vi "shake it.vi"(4 "cursor bracket : fragment 2":refnum<vi>, 5 "modify if out of window?":bool=TRUE, 6 "cursor bracket: All, data window 2":refnum<vi>, 7 "Plot: All":refnum<vi>, 8 "follow the peak Con":T1={"factor"=3.0, "omega ?"=TRUE, "gamma ?"=TRUE, "max (kHz)"=3.0, "is clean"=TRUE, "acceptance"=0.3, "history - length"=10}, 9 "search attempts":i32=4, 10 "peak close to center -- factor":dbl=0.3, 11 "lorentzian":T3={"Amplitude"=0.005126003617902175, "omega(0)"=2152.184993711879, "Gamma"=1.6893036092699798, "phase"=-0.5171067718590723, "Q"=1274.0072192481316, "Norm  Ampl"=0.7704795248463377, "z (inf)"=0.18381077367248932+0.35479358908517594i, "4corners"={"z (-pi/2)"=0.35479358908517594-0.2671441070058228i, "z(inf)"=0.18381077367248932+0.35479358908517594i, "z (pi/2)"=-0.4381269224185094+0.18381077367248932i, "z center"=-0.04166666666666674-0.04166666666666674i, "z(0)"=-0.2671441070058228-0.4381269224185094i, "radius"=0.4560929844809216}} {"z (inf)" format="%#9_9f"; "Q" format="%#9_9f"; "phase" format="%#9_9f"; "Gamma" format="%#9_9f"; "omega(0)" format="%#9_9f"}) -> (0 "Boolean":bool, 1 "worth trying":bool, 2 "in range?":bool=TRUE, 3 "lorentzian out":T3={"Amplitude"=0.005126003617902175, "omega(0)"=2152.184993711879, "Gamma"=1.6893036092699798, "phase"=-0.5171067718590723, "Q"=1274.0072192481316, "Norm  Ampl"=0.7704795248463377, "z (inf)"=0.18381077367248932+0.35479358908517594i, "4corners"={"z (-pi/2)"=0.35479358908517594-0.2671441070058228i, "z(inf)"=0.18381077367248932+0.35479358908517594i, "z (pi/2)"=-0.4381269224185094+0.18381077367248932i, "z center"=-0.04166666666666674-0.04166666666666674i, "z(0)"=-0.2671441070058228-0.4381269224185094i, "radius"=0.4560929844809216}} {"z (inf)" format="%#9_9f"; "Q" format="%#9_9f"; "phase" format="%#9_9f"; "Gamma" format="%#9_9f"; "omega(0)" format="%#9_9f"})   [LabVIEW 2015]
uses:
  lorentzian.ctl
  circle corners.ctl
  cursor winow.ctl
  follow the peak control.ctl
  cursor window action.ctl
panel:
  in  "cursor bracket in":T2={"left"=2044.0881763527054, "right "=2126.7657992565055, "center"=2085.4269878046052, "window"=82.67762290380006, "cursors"=[], "relative"=0, "absolute"=0, "fixed vertical offset"=2421.6740576496672, "vertical offset"=2421.6740576496672, "skew"=2421.6740576496672, "default window frac"=2421.6740576496672, "kind"=enum."fancy", "skew.left"=2.0, "skew.right"=0.0, "Plot ref"=refnum, "wing order"=enum."back"}
  in  "follow the peak is clean -- out":bool
  out "attempts to success":i32
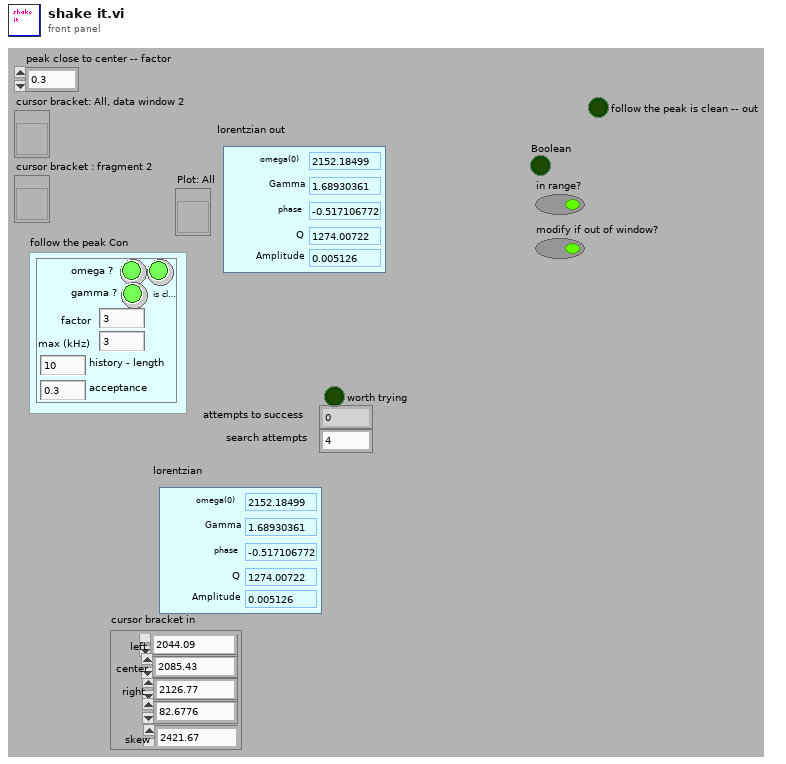
[diagram p1: front panel]
types:
  T1 = typedef "follow the peak control.ctl" = cluster{"factor":dbl, "omega ?":bool, "gamma ?":bool, "max (kHz)":dbl, "is clean":bool, "acceptance":dbl, "history - length":i32}
  T2 = typedef "cursor winow.ctl" = cluster{"left":dbl, "right ":dbl, "center":dbl, "window":dbl, "cursors":i32[], "relative":i32, "absolute":i32, "fixed vertical offset":dbl, "vertical offset":dbl, "skew":dbl, "default window frac":dbl, "kind":enum16{"symmetric", "skewed", "fancy"}, "skew.left":dbl, "skew.right":dbl, "Plot ref":refnum<vi>, "wing order":enum16{"forw", "back"}}
  T3 = typedef "lorentzian.ctl" = cluster{"Amplitude":dbl, "omega(0)":dbl, "Gamma":dbl, "phase":dbl, "Q":dbl, "Norm  Ampl":dbl, "z (inf)":cdb, "4corners":T4}
  T4 = typedef "circle corners.ctl" = cluster{"z (-pi/2)":cdb, "z(inf)":cdb, "z (pi/2)":cdb, "z center":cdb, "z(0)":cdb, "radius":dbl}
  T5 = typedef "cursor window action.ctl" = enum16{"balance", "h. offset change", "cursor moves", "change center", "change window", "init", "check", "reset", "set y to middle", "idle", "-write all Y", "-write left.X", "-write center.X", "-write right.X", "-write all X", "-change center", "-change window", "-change skew", "-read cursor 2", "-read cursor 1", "-read cursor 0", "-read all cursors", "-reset", "-read plot scale", "-set y to middle", "-Q: center.Y is visible", "-Q: window is visible", "-parse center.Y", "-right left from center", "-left move", "-right move", "-set center.Y", "-empty", "-set cursors to default", "-check", "-write center.Y", "-copy cursor 1", "-copy cursor 0", "-copy cursor 2", "move right", "move left", "shrink", "broaden", "skew up", "skew down", "-write plot scale", "zoom X", "change cen&win", "zoom to all data"}
  T6 = enum16{"normal", "alert", "fuzzy", "interesting", "boring", "colored"}
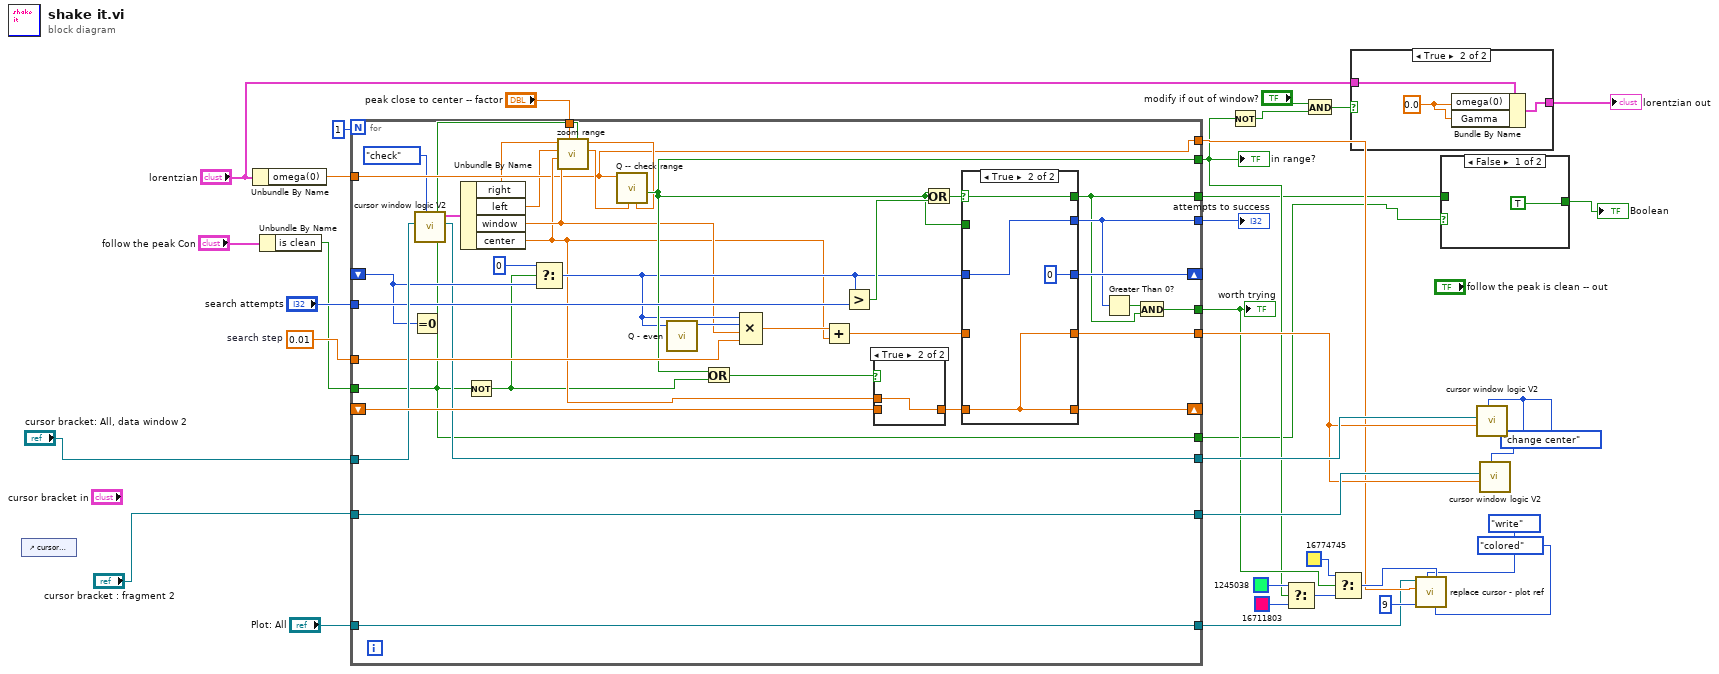
[diagram p0: block diagram]
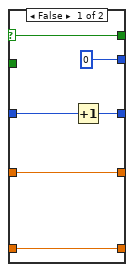
[diagram p5: hidden frame]
diagram:
  w5 = cursor_window_action."change center" ("cursor window action")
  w30 = 0.01  # search step
  n1 = control-ref of="cursor bracket in"() -> ()  [unwired: 1 out]
  n2 = Unbundle By Name("lorentzian") -> ("omega(0)"=w33:dbl)
  n3 = Unbundle By Name("follow the peak Con") -> ("is clean"=w1:bool)
  n4 = for {
    N: 1 -> [_]
    shift-right: [w72] -> _
    shift-left: _ -> [w51]
    shift-right: [w70] -> _
    shift-left: _ -> [w69]
    tunnel: "Plot: All" -> [w47]
    tunnel: "cursor bracket: All, data window 2" -> [w62]
    tunnel: w33 -> [w42]
    tunnel: [w57] -> w6
    tunnel: "cursor bracket : fragment 2" -> [w49]
    tunnel: [w58] -> w32
    tunnel: [w54] -> w10
    tunnel: "search attempts" -> [w61]
    tunnel: w30 -> [w60]
    tunnel: [w56] -> w13
    tunnel: w1 -> [w40]
    tunnel: [w50] -> w24
    tunnel: [w49] -> w23
    tunnel: [w48] -> w22
    tunnel: [w42] -> w12
    tunnel: [w47] -> w11
    tunnel: [w40] -> w8
    tunnel: "peak close to center -- factor" -> [w41]
    n5 = Equal To 0?(x=w51) -> ()  [unwired: 1 out]
    n6 = call "cursor window logic V2.vi"("cursor window action"=cursor_window_action."check", "cursor window in"=w62) -> (2:"cursor window out"=w50:refnum<vi>, 3:"cursor window out"=w68:T2)  [unwired: 8 in]
    n7 = Unbundle By Name(w68) -> ("right"=w39:dbl, "left"=w38:dbl, "window"=w46:dbl, "center"=w45:dbl)
    n8 = Not(x=w40) -> (.not. x?=w37:bool)
    n9 = Select(t=0 ("interval"), s=w37, f=w51) -> (s? t:f=w53:i32)
    n10 = call "zoom range.vi"("zoom?"=w40, "factor"=w41, "window"=w46, "center"=w45, "left"=w38, "right"=w39) -> ("left out"=w44:dbl, "right out"=w43:dbl)  [unwired: 2 in, 2 out]
    n11 = call "Q -- check range.vi"("upper"=w43, "lower"=w44, "number"=w42) -> ("in range?"=w54:bool)  [unwired: 4 in, 4 out]
    n12 = call "Q - even.vi"("Numeric"=w53) -> ("saw"=w66:i32)  [unwired: 9 in, 1 out]
    n13 = Or(x=w54, y=w37) -> (x .or. y?=w55:bool)
    n14 = Compound Arithmetic op=MULTIPLY(w53, w66, w46, w60) -> (w67:dbl)
    n15 = Add(x=w67, y=w45) -> (x+y=w71:dbl)
    n16 = Greater?(x=w53, y=w61) -> (0:w64:bool)
    n17 = case shown="True" w55 {
      tunnel: [w73 w74] -> w63
      tunnel: w45 -> [_ w74]
      tunnel: w69 -> [w73 _]
      frame False {
      }
      frame True {
      }
    }
    n18 = Or(x=w54, y=w64) -> (x .or. y?=w65:bool)
    n19 = case shown="True" w65 {
      selector: w65 -> [w77 w83]
      tunnel: [w79 0 ("interval")] -> w72
      tunnel: w53 -> [w80 w82]
      tunnel: w71 -> [w75 _]
      tunnel: [w78 w81] -> w70
      tunnel: w63 -> [w78 w81]
      tunnel: w54 -> [_ _]
      tunnel: [w77 w83] -> w57
      tunnel: [0 ("interval") w82] -> w58
      tunnel: [w75 w81] -> w48
      frame False {
        n20 = Increment(x=w80) -> (x+1=w79:i32)
      }
      frame True {
      }
    }
    n21 = Greater Than 0?(x=w58) -> (x > 0?=w59:bool)
    n22 = And(x=w59, y=w57) -> (x .and. y?=w56:bool)
  }
  "attempts to success" <- w32
  "in range?" <- w10
  "worth trying" <- w13
  n23 = Not(x=w10) -> (.not. x?=w29:bool)
  n24 = Select(t=u32 1245038, s=w10, f=u32 16711803) -> (s? t:f=w20:u32)
  n25 = And(x="modify if out of window?", y=w29) -> (x .and. y?=w25:bool)
  n26 = Select(t=u32 16774745, s=w13, f=w20) -> (s? t:f=w21:u32)
  n27 = case shown="True" w25 {
    tunnel: "lorentzian" -> [w85 w88]
    tunnel: [w85 w87] -> w26
    frame False {
    }
    frame True {
      w86 = 0.0
      n28 = Bundle By Name(cluster=w88, "omega(0)"=w86, "Gamma"=w86) -> (w87:T3)
    }
  }
  "lorentzian out" <- w26
  n29 = call "replace cursor - plot ref.vi"("cursor state"=T6."colored", "Color Box"=w21, "action"=enum16{"", "read", "write"}."write" ("Enum"), "cursor index"=9, "new X"=w12, "Plot ref in"=w11) -> ()  [unwired: 3 in, 3 out]
  n30 = case shown="False" w8 {
    tunnel: [TRUE w90] -> w7
    tunnel: w6 -> [_ w90]
    frame False {
    }
    frame True {
    }
  }
  "Boolean" <- w7
  n31 = call "cursor window logic V2.vi"("cursor window action"=w5, "center"=w22, "cursor window in"=w24) -> ()  [unwired: 7 in, 2 out]
  n32 = call "cursor window logic V2.vi"("cursor window action"=w5, "center"=w22, "cursor window in"=w23) -> ()  [unwired: 7 in, 2 out]
